vi "multistep.vi"(0 "VISA resource name 2":refnum<visa-resource-name>, 1 "y":sgl=5.0, 5 "Numeric 5":sgl=-10.0, 7 "Numeric 2":sgl=0.1, 9 "Numeric 3":sgl=0.1, 11 "error out 2":errorcluster, 12 "new element/subarray":i32=1, 13 "millisecond multiple":u32=5) -> (4 "VISA resource name 3":refnum<visa-resource-name>, 8 "Numeric 4":i32, 15 "error out 3":errorcluster)   [LabVIEW 2017]
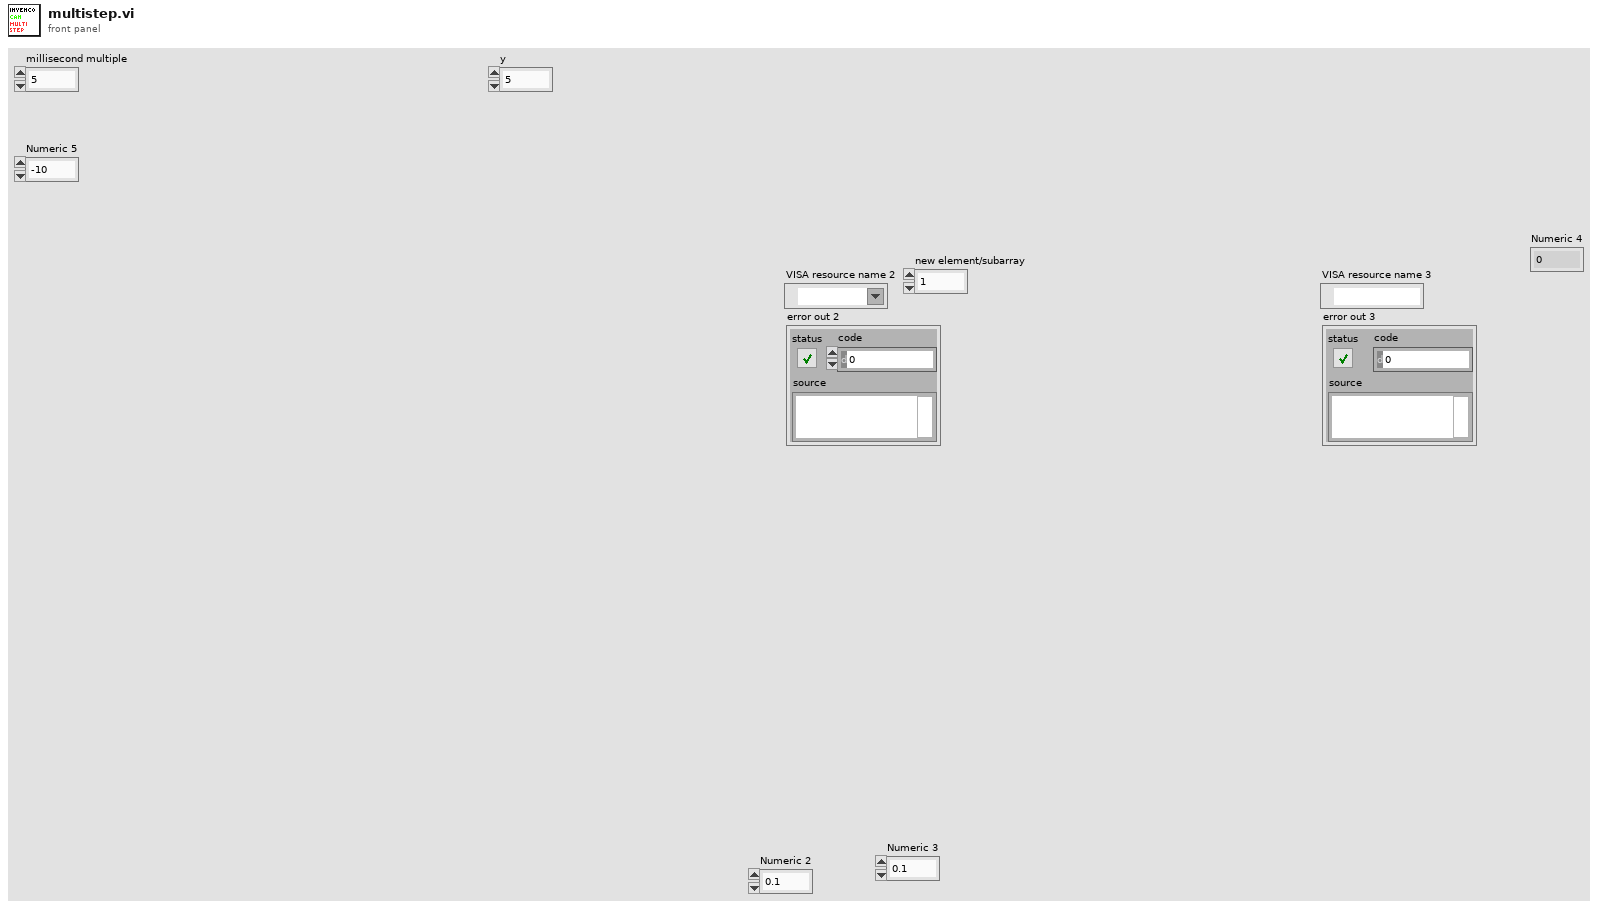
[diagram p1: front panel]
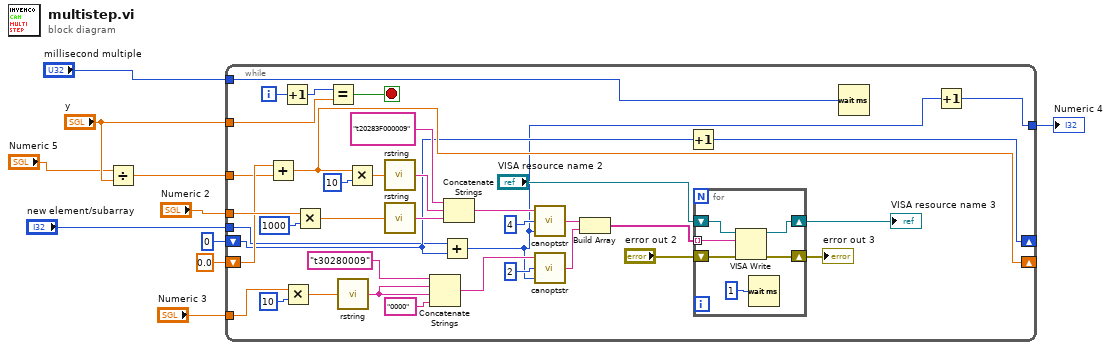
[diagram p0: block diagram]
diagram:
  n1 = Divide(x="Numeric 5", y="y") -> (x/y=w6:sgl)
  n2 = while {
    tunnel: "new element/subarray" -> [w17]
    shift-right: [w25] -> _
    shift-left: 0 -> [w18]
    tunnel: "Numeric 3" -> [w24]
    tunnel: "Numeric 2" -> [w23]
    tunnel: w6 -> [w20]
    shift-right: [w19] -> _
    shift-left: 0.0 -> [w21]
    tunnel: [w12] -> w4
    tunnel: "y" -> [w14]
    tunnel: "millisecond multiple" -> [w11]
    i -> [w16]
    stop <- w22 stop-if-true
    n3 = Add(x=w21, y=w20) -> (x+y=w19:dbl)
    n4 = Increment(x=w16) -> (x+1=w15:i32)
    n5 = Multiply(x=w24, y=i16 10) -> (x*y=w32:sgl)
    n6 = Multiply(x=w23, y=i16 1000) -> (x*y=w34:sgl)
    n7 = Equal?(x=w15, y=w14) -> (x = y?=w22:bool)
    n8 = call "rstring.vi"("number"=w32) -> ("concatenated string"=w29:string)
    n9 = Multiply(x=w19, y=i16 10) -> (x*y=w37:dbl)
    n10 = call "rstring.vi"("number"=w37) -> ("concatenated string"=w36:string)
    n11 = call "rstring.vi"("number"=w34) -> ("concatenated string"=w33:string)
    n12 = Concatenate Strings("t30280009", w29, w29, "0000" ("string")) -> (w26:string)
    n13 = Add(x=w17, y=w18) -> (x+y=w13:i32)
    n14 = Concatenate Strings("t20283F000009", w36, w33) -> (w27:string)
    n15 = call "canoptstr.vi"("new element/subarray"=w13, "index"=4, "String 2"=w27) -> ("String"=w43:string)
    n16 = call "canoptstr.vi"("new element/subarray"=w13, "index"=2, "String 2"=w26) -> ("String"=w44:string)
    n17 = Build Array(w43, w44) -> (w40:string[])
    n18 = Increment(x=w18) -> (x+1=w25:i32)
    n19 = for {
      tunnel: w40 -> [w50] mode=indexing
      shift-right: [w52] -> w48
      shift-left: "VISA resource name 2" -> [w54]
      shift-right: [w51] -> w47
      shift-left: "error out 2" -> [w53]
      n20 = VISA Write(VISA resource name=w54, write buffer=w50, error in (no error)=w53) -> (VISA resource name out=w52:refnum<visa-resource-name>, error out=w51:errorcluster)  [unwired: 1 out]
      n21 = Wait (ms)(milliseconds to wait=u32 1 ("millisecond multiple")) -> ()  [unwired: 1 out]
    }
    "VISA resource name 3" <- w48
    "error out 3" <- w47
    n22 = Wait (ms)(milliseconds to wait=w11) -> ()  [unwired: 1 out]
    n23 = Increment(x=w13) -> (x+1=w12:i32)
  }
  "Numeric 4" <- w4
